vi "Build Internal State String.vi"(5 "State":string, 7 "Arguments (\"\")":string, 9 ">> Response Source Message >>":T1, 11 "Source (\"\")":string) -> (6 "State with Arguments":string)   [LabVIEW 2020, in "Communicable State Machine.lvlib"]
doc: "Build a state string that contains arguments for the CSM.\n\n<b>Inputs:</b>s\n - <b>State</b>: The State or message string\n - <b>Arguments (\"\")</b>: The argument for <b>State</b>\n - <b>Arg-State (\"\")</b>: Why this message is sent here\n - <b>Source (\"\")</b>: Who sent this message here\n\n<b>Outputs:</b>\n - <b>State with Arguments</b>: String stands for state with arguments"
uses:
  Communicable State Machine.lvlib
  _CSM_Response Source Message.ctl
  CSM - Make String Arguments Safe.vi
  CSM - Keywords.vi
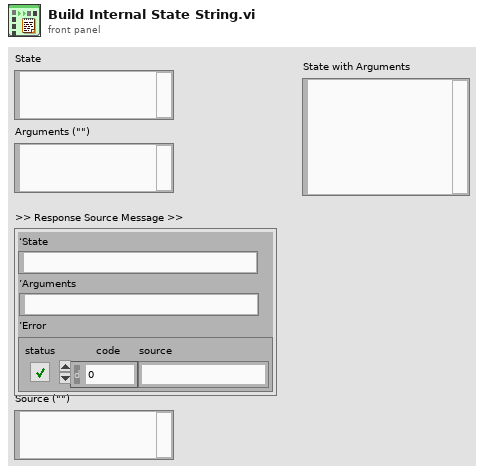
[diagram p1: front panel]
types:
  T1 = typedef "Communicable State Machine.lvlib/_CSM_Response Source Message.ctl" = cluster{"‘State":string, "’Arguments":string, "’Error":errorcluster}
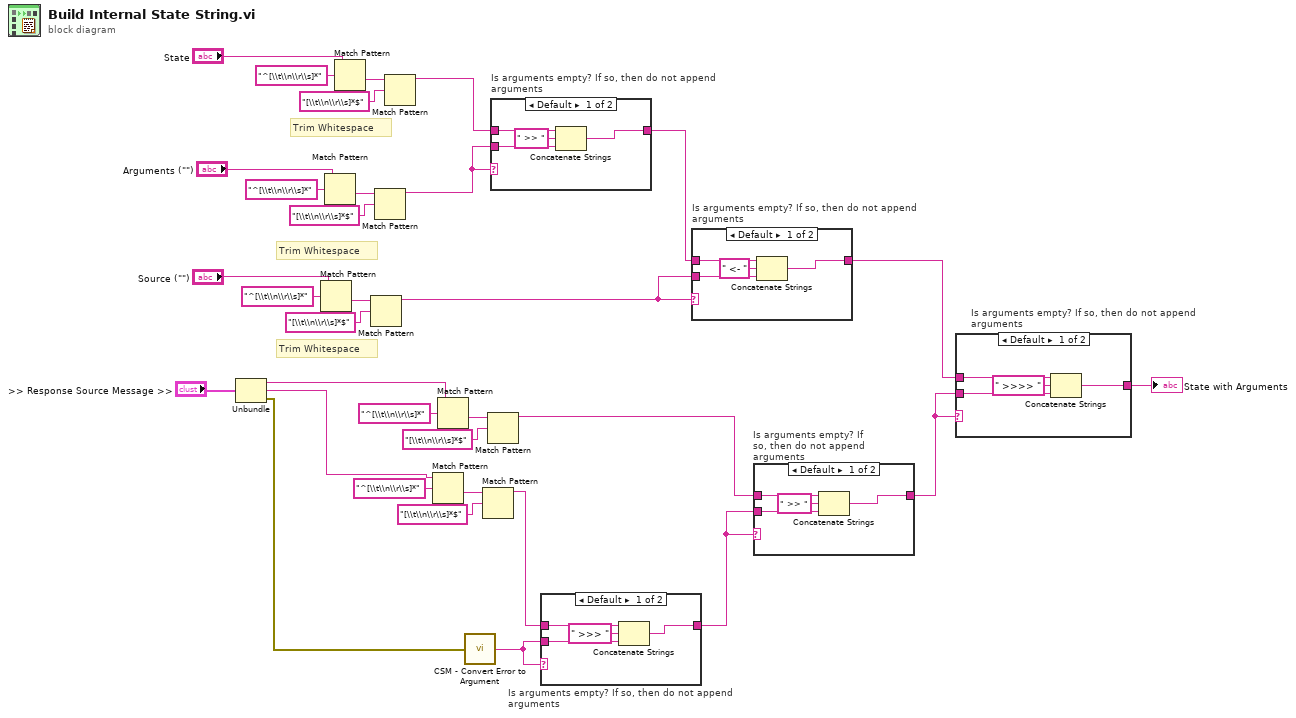
[diagram p0: block diagram]
diagram:
  # "Trim Whitespace"
  # "Trim Whitespace"
  # "Trim Whitespace"
  n1 = Unbundle(">> Response Source Message >>") -> ("‘State"=w11:string, "’Arguments"=w7:string, "’Error"=w5:errorcluster)
  n2 = Match Pattern(string="Source (\"\")", regular expression="^[\\t\\n\\r\\s]*") -> (after substring=w22:string)  [unwired: 1 in, 3 out]
  n3 = Match Pattern(string="Arguments (\"\")", regular expression="^[\\t\\n\\r\\s]*") -> (after substring=w27:string)  [unwired: 1 in, 3 out]
  n4 = Match Pattern(string="State", regular expression="^[\\t\\n\\r\\s]*") -> (after substring=w32:string)  [unwired: 1 in, 3 out]
  n5 = Match Pattern(string=w22, regular expression="[\\t\\n\\r\\s]*$") -> (before substring=w19:string)  [unwired: 1 in, 3 out]
  n6 = Match Pattern(string=w27, regular expression="[\\t\\n\\r\\s]*$") -> (before substring=w24:string)  [unwired: 1 in, 3 out]
  n7 = Match Pattern(string=w32, regular expression="[\\t\\n\\r\\s]*$") -> (before substring=w29:string)  [unwired: 1 in, 3 out]
  n8 = Match Pattern(string=w7, regular expression="^[\\t\\n\\r\\s]*") -> (after substring=w9:string)  [unwired: 1 in, 3 out]
  n9 = Match Pattern(string=w11, regular expression="^[\\t\\n\\r\\s]*") -> (after substring=w17:string)  [unwired: 1 in, 3 out]
  n10 = call "CSM - Convert Error to Argument.vi"("error in (no error)"=w5) -> ("Arguments"=w4:string)  [unwired: 4 in]
  n11 = Match Pattern(string=w9, regular expression="[\\t\\n\\r\\s]*$") -> (before substring=w2:string)  [unwired: 1 in, 3 out]
  n12 = Match Pattern(string=w17, regular expression="[\\t\\n\\r\\s]*$") -> (before substring=w6:string)  [unwired: 1 in, 3 out]
  n13 = case "Is arguments empty? If so, then do not append arguments" shown="Default" w24 {
    tunnel: [w34 w38] -> w14
    tunnel: w29 -> [w37 w38]
    tunnel: w24 -> [w35 _]
    frame Default {
      n14 = Concatenate Strings(w37, " >> " ("string"), w35) -> (w34:string)
    }
    frame "" {
    }
  }
  n15 = case "Is arguments empty? If so, then do not append arguments" shown="Default" w4 {
    tunnel: [w39 w43] -> w1
    tunnel: w2 -> [w42 w43]
    tunnel: w4 -> [w40 _]
    frame Default {
      n16 = Concatenate Strings(w42, " >>> " ("string"), w40) -> (w39:string)
    }
    frame "" {
    }
  }
  n17 = case "Is arguments empty? If so, then do not append arguments" shown="Default" w19 {
    tunnel: [w44 w48] -> w13
    tunnel: w14 -> [w47 w48]
    tunnel: w19 -> [w45 _]
    frame Default {
      n18 = Concatenate Strings(w47, " <- " ("string"), w45) -> (w44:string)
    }
    frame "" {
    }
  }
  n19 = case "Is arguments empty? If so, then do not append arguments" shown="Default" w1 {
    tunnel: [w49 w53] -> w3
    tunnel: w6 -> [w52 w53]
    tunnel: w1 -> [w50 _]
    frame Default {
      n20 = Concatenate Strings(w52, " >> " ("string"), w50) -> (w49:string)
    }
    frame "" {
    }
  }
  n21 = case "Is arguments empty? If so, then do not append arguments" shown="Default" w3 {
    tunnel: [w55 w58] -> w12
    tunnel: w13 -> [w57 w58]
    tunnel: w3 -> [w56 _]
    frame Default {
      n22 = Concatenate Strings(w57, " >>>> " ("string"), w56) -> (w55:string)
    }
    frame "" {
    }
  }
  "State with Arguments" <- w12
